vi "State History.vi"(7 "Current State":string) -> (3 "History":string)   [LabVIEW 2016, in "Instrument.lvclass"]
uses:
  Instrument.lvclass
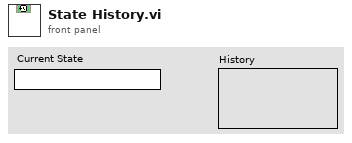
[diagram p1: front panel]
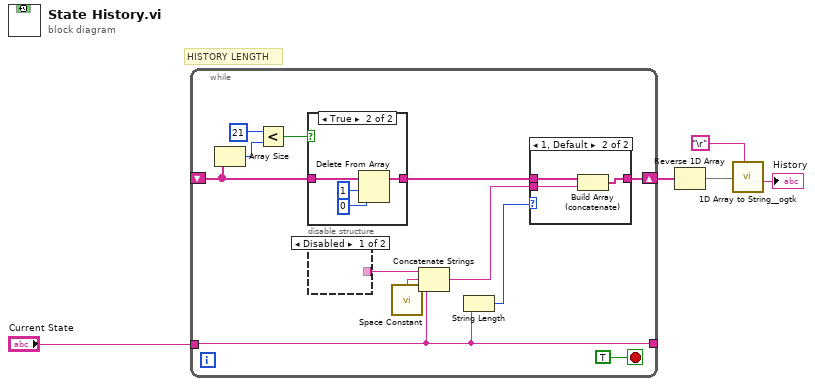
[diagram p0: block diagram]
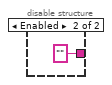
[diagram p2: hidden frame]
diagram:
  # "HISTORY LENGTH"
  n1 = while {
    tunnel: "Current State" -> [w12]
    tunnel: [w12] -> _
    shift-right: [w13] -> w3
    shift-left: _ -> [w6]
    stop <- TRUE stop-if-true
    n2 = Array Size(array=w6) -> (size(s)=w16:i32)
    n3 = Less?(x=21 ("length"), y=w16) -> (x < y?=w9:bool)
    n4 = case shown="True" w9 {
      tunnel: w6 -> [w23 w24]
      tunnel: [w23 w26] -> w17
      frame False {
      }
      frame True {
        n5 = Delete From Array(array=w24, length=1, index=0) -> (array with subset deleted=w26:string[])  [unwired: 1 out]
      }
    }
    n6 = disable-structure shown="Disabled" {
      disable-tunnel: [_ "" ("Spinner Out")] -> w11
      frame Disabled {
      }
      frame Enabled {
      }
    }
    n7 = call <vilib>:"Space Constant.vi"() -> ("String"=w10:string)
    n8 = Concatenate Strings(w11, w10, w12) -> (w8:string)
    n9 = String Length(string=w12) -> (length=w7:i32)
    n10 = case shown="1, Default" w7 {
      tunnel: w17 -> [w19 w21]
      tunnel: [w19 w22] -> w13
      tunnel: w8 -> [_ w20]
      frame 0 {
      }
      frame 1, Default {
        n11 = Build Array (concatenate)(w21, w20) -> (w22:string[])
      }
    }
  }
  n12 = Reverse 1D Array(array=w3) -> (reversed array=w2:string[])
  n13 = call <userlib>:"1D Array to String__ogtk.vi"("delimiter (Tab)"="\r", "Array of Strings"=w2) -> ("delimited string"=→"History":string)  [unwired: 9 in]
